vi "QT_Call_Win.vi"(0 "QT Ref In":T11, 1 "Frame Grabber Settings":T15={"Name"="", "Digitizer"=0, "Input"=0, "Width"=0, "Height"=0, "Input format"=enum."PAL", "Frame rate"=0.0, "Reserved"=0, "Dialogs"=0} {"Frame rate" format="%#1_6g"; "Dialogs" format="%.0b"}, 2 "Compression Settings":T14 {"Dialogs" format="%.0b"; "Comp. Quality" format="%.0x"; "Codec" format="%.0x"}, 3 "Movie Settings":T10 {"Dialogs" format="%.0b"}, 4 "Image in":T5 {"Dialogs" format="%.0b"}, 5 "Sound in":T4 {"Rate" format="%x"}, 6 "Selector":T16, 7 "Video Settings in":T3={"Color format"=1, "Hue"=0.0, "Saturation"=0.0, "Brightness"=0.0, "Contrast"=0.0, "Sharpness"=0.0, "Black Level"=0.0, "White Level"=0.0, "Options"=0, "Dialogs"=0} {"Dialogs" format="%.0b"; "Color format" items=["Black & White (8 bits)", "RGB (24 bits)", "RGBx (32 bits)", "RGBA (32bits)", "RGB B&W (32 bits)", "HSI (24 bits)", "HSIx (32 bits)", "HSI B&W (32 bits)"]; "Brightness" format="%.2f"; "Contrast" format="%.2f"; "Sharpness" format="%.2f"; "Black Level" format="%.2f"; "White Level" format="%.2f"; "Saturation" format="%.2f"; "Hue" format="%.2f"}, 8 "Private":T6, 9 "Effect":T9 {"Matrix" format="%.2f"}, 11 "File Settings":T13 {"Dialogs" format="%.0b"}) -> (12 "Info Out":T12, 13 "Video Settings out":T3={"Color format"=1, "Hue"=0.0, "Saturation"=0.0, "Brightness"=0.0, "Contrast"=0.0, "Sharpness"=0.0, "Black Level"=0.0, "White Level"=0.0, "Options"=0, "Dialogs"=0} {"Dialogs" format="%.0b"; "Color format" items=["Black & White (8 bits)", "RGB (24 bits)", "RGBx (32 bits)", "RGBA (32bits)", "RGB B&W (32 bits)", "HSI (24 bits)", "HSIx (32 bits)", "HSI B&W (32 bits)"]; "Brightness" format="%.2f"; "Contrast" format="%.2f"; "Sharpness" format="%.2f"; "Black Level" format="%.2f"; "White Level" format="%.2f"; "Saturation" format="%.2f"; "Hue" format="%.2f"}, 14 "QT Ref Out":T11, 16 "Movie info":T7 {"Tracks"."Rate" format="%.2f"}, 17 "QT Info":T1 {"Digitizers"."In Flags" format="%.0b"; "Digitizers"."Out Flags" format="%.0b"; "Digitizers"."Inputs" items=["Composite", "S-Video", "RGB", "RGB Synch", "YUV", "YUV Synch", "TV Tuner", "sdiln"]; "CIN rev ID" format="%.2f"}, 18 "Image/Movie Out":T5 {"Dialogs" format="%.0b"}, 19 "Sound out":T4 {"Rate" format="%x"})   [LabVIEW 2024]
uses:
  <userlib>/ImageProcessing/QTLIB_2595_LV86/QT_FrameGrabber.ctl
  <userlib>/ImageProcessing/QTLIB_2595_LV86/QT_Video.ctl
  <userlib>/ImageProcessing/QTLIB_2595_LV86/QT_Movie.ctl
  <userlib>/ImageProcessing/QTLIB_2595_LV86/QT_Compression.ctl
  <userlib>/ImageProcessing/QTLIB_2595_LV86/QT_Private.ctl
  <userlib>/ImageProcessing/QTLIB_2595_LV86/QT_Effect.ctl
  <userlib>/ImageProcessing/QTLIB_2595_LV86/QT_Image.ctl
  <userlib>/ImageProcessing/QTLIB_2595_LV86/QT_Sound.ctl
  <userlib>/ImageProcessing/QTLIB_2595_LV86/QT_File.ctl
  <userlib>/ImageProcessing/QTLIB_2595_LV86/QT_Digitizer.ctl
  <userlib>/ImageProcessing/QTLIB_2595_LV86/QT_Info.ctl
  <userlib>/ImageProcessing/QTLIB_2595_LV86/QT_Selector.ctl
  <userlib>/ImageProcessing/QTLIB_2595_LV86/QT_Ref.ctl
  <userlib>/ImageProcessing/QTLIB_2595_LV86/QT_Track.ctl
  <userlib>/ImageProcessing/QTLIB_2595_LV86/QT_MovieInfo.ctl
  <userlib>/ImageProcessing/QTLIB_2595_LV86/QT_ErrInfo.ctl
panel:
  # "[0,0] [0,1]  [0,2] [1,0].. [2,2]"
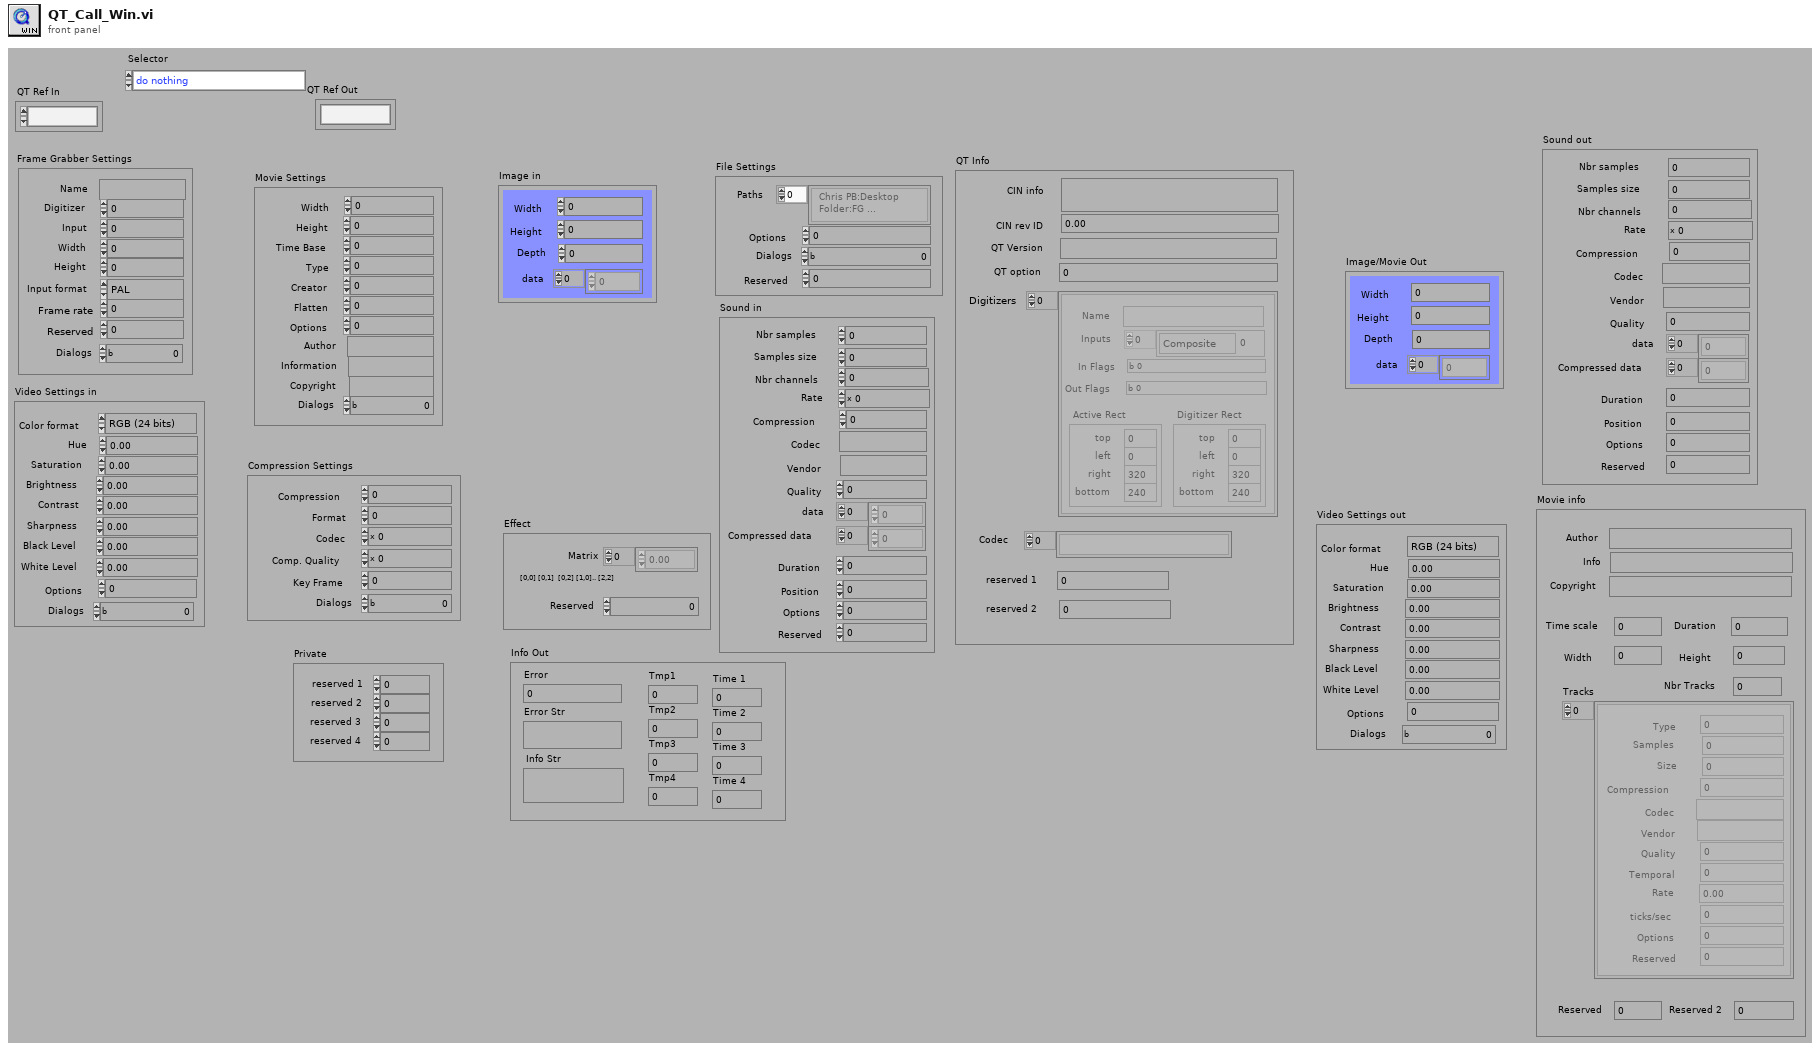
[diagram p1: front panel]
types:
  T1 = typedef "QT_Info.ctl" = cluster{"CIN info":string, "CIN rev ID":dbl, "QT Version":string, "QT option":i32, "Digitizers\n":T2[], "Codec":string[], "reserved 1":i32, "reserved 2":i32}
  T2 = typedef "QT_Digitizer.ctl" = cluster{"Name":string, "Inputs":i32[], "In Flags":i32, "Out Flags":i32, "Digitizer Rect":cluster{"top":i32, "left":i32, "right":i32, "bottom":i32}, "Active Rect":cluster{"top":i32, "left":i32, "right":i32, "bottom":i32}}
  T3 = typedef "QT_Video.ctl" = cluster{"Color format":u32, "Hue":dbl, "Saturation":dbl, "Brightness":dbl, "Contrast":dbl, "Sharpness":dbl, "Black Level":dbl, "White Level":dbl, "Options":i32, "Dialogs":u32}
  T4 = typedef "QT_Sound.ctl" = cluster{"Nbr samples":i32, "Samples size":i32, "Nbr channels":i32, "Rate ":i32, "Compression":i32, "Codec":string, "Vendor":string, "Quality":i32, "data":i16[], "Compressed data":u8[], "Duration":i32, "Position":i32, "Options":i32, "Reserved":i32}
  T5 = typedef "QT_Image.ctl" = cluster{"Width":i32, "Height":i32, "Depth":i32, "data":u8[], "Compressed data":u8[], "Color table":u32[], "Duration":i32, "Options":i32, "Timestamp":i32, "ID":i32, "Reserved":i32, "Dialogs":u32}
  T6 = typedef "QT_Private.ctl" = cluster{"reserved 1":i32, "reserved 2":i32, "reserved 3":i32, "reserved 4":i32}
  T7 = typedef "QT_MovieInfo.ctl" = cluster{"Author":string, "Info":string, "Copyright":string, "Time scale":i32, "Duration":i32, "Width":i32, "Height":i32, "Nbr Tracks":i32, "Tracks":T8[], "Reserved":i32, "Reserved 2":i32}
  T8 = typedef "QT_Track.ctl" = cluster{"Type":i32, "Samples":i32, "Size":i32, "Compression":i32, "Codec":string, "Vendor":string, "Quality":i32, "Temporal":i32, "Rate ":dbl, "ticks/sec":i32, "Options":i32, "Reserved":i32}
  T9 = typedef "QT_Effect.ctl" = cluster{"Reserved":i32, "Matrix":dbl[]}
  T10 = typedef "QT_Movie.ctl" = cluster{"Width":i32, "Height":i32, "Time Base":i32, "Type":i32, "Creator":i32, "Flatten":i32, "Options":i32, "Author":string, "Information":string, "Copyright":string, "Dialogs":u32}
  T11 = typedef "QT_Ref.ctl" = refnum<k1>
  T12 = typedef "QT_ErrInfo.ctl" = cluster{"Error":i32, "Error Str":string, "Info Str":string, "Tmp1":i32, "Tmp2":i32, "Tmp3":i32, "Tmp4":i32, "Time 1":i32, "Time 2":i32, "Time 3":i32, "Time 4":i32}
  T13 = typedef "QT_File.ctl" = cluster{"Paths":string[], "Options":i32, "Dialogs":u32, "Reserved":i32}
  T14 = typedef "QT_Compression.ctl" = cluster{"Compression":i32, "Format":i32, "Codec":i32, "Comp. Quality":i32, "Key Frame":i32, "Dialogs":u32}
  T15 = typedef "QT_FrameGrabber.ctl" = cluster{"Name":string, "Digitizer":i32, "Input":i32, "Width":i32, "Height":i32, "Input format":enum32{"NTSC", "PAL", "Secam"}, "Frame rate":dbl, "Reserved":i32, "Dialogs":u32}
  T16 = typedef "QT_Selector.ctl" = enum32{"do nothing", "Get all Sources", "Get Source info", "Open Image", "Save Image to File", "Effect", "Close", "SG Grab", "Compress in Memory", "Decompress to Memory", "New Movie", "Open Movie", "Add Frame", "Get Frame", "Close Movie", "Get QT & CIN info", "SG init", "SG Close", "Open sound file", "Close sound file", "Read sound data", "Write sound data", "Import sound", "Export sound", "Add sound to movie", "Get sound from movie", "reserved", "reserved 1", "reserved 2"}
  T17 = cluster{"Color format":u32, "Hue":dbl, "Saturation":dbl, "Brightness":dbl, "Contrast":dbl, "Sharpness":dbl, "Black Level":dbl, "White Level":dbl, "Options":i32, "Dialogs":u32}
  T18 = cluster{"Author":string, "Info":string, "Copyright":string, "Time scale":i32, "Duration":i32, "Width":i32, "Height":i32, "Nbr Tracks":i32, "Tracks":cluster{"Type":i32, "Samples":i32, "Size":i32, "Compression":i32, "Codec":string, "Vendor":string, "Quality":i32, "Temporal":i32, "Rate ":dbl, "ticks/sec":i32, "Options":i32, "Reserved":i32}[], "Reserved":i32, "Reserved 2":i32}
  T19 = cluster{"Width":i32, "Height":i32, "Depth":i32, "data":u8[], "Compressed data":u8[], "Color table":u32[], "Duration":i32, "Options":i32, "Timestamp":i32, "ID":i32, "Reserved":i32, "Dialogs":u32}
  T20 = cluster{"Nbr samples":i32, "Samples size":i32, "Nbr channels":i32, "Rate ":i32, "Compression":i32, "Codec":string, "Vendor":string, "Quality":i32, "data":i16[], "Compressed data":u8[], "Duration":i32, "Position":i32, "Options":i32, "Reserved":i32}
  T21 = cluster{"Error":i32, "Error Str":string, "Info Str":string, "Tmp1":i32, "Tmp2":i32, "Tmp3":i32, "Tmp4":i32, "Time 1":i32, "Time 2":i32, "Time 3":i32, "Time 4":i32}
  T22 = cluster{"CIN info":string, "CIN rev ID":dbl, "QT Version":string, "QT option":i32, "Digitizers\n":cluster{"Name":string, "Inputs":i32[], "In Flags":i32, "Out Flags":i32, "Digitizer Rect":cluster{"top":i32, "left":i32, "right":i32, "bottom":i32}, "Active Rect":cluster{"top":i32, "left":i32, "right":i32, "bottom":i32}}[], "Codec":string[], "reserved 1":i32, "reserved 2":i32}
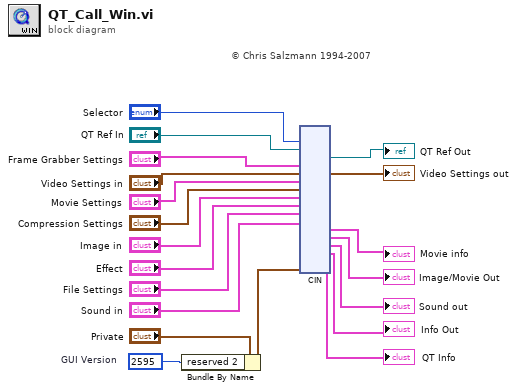
[diagram p0: block diagram]
diagram:
  w1 = 2595  # GUI Version
  # "© Chris Salzmann 1994-2007"
  n1 = Bundle By Name(cluster="Private", "reserved 2"=w1) -> (w3:T6)
  n2 = cin("Selector", "QT Ref In", "Frame Grabber Settings", "Video Settings in", "Movie Settings", "Compression Settings", "Image in", "Effect", "File Settings", "Sound in", w3) -> (→"QT Ref Out":refnum<k1>, →"Video Settings out":T17, →"Movie info":T18, →"Image/Movie Out":T19, →"Sound out":T20, →"Info Out":T21, →"QT Info":T22)  [unwired: 16 in]
